vi "error_example.vi"() -> ()   [LabVIEW 2023, in "Error Handling Interface.lvlib" / "Error.lvclass"]
doc: "Demonstrates how to construct an error object and retrieve the log item from the class"
uses:
  Error.lvclass
  <vilib>/ActorFramework/Actor/Actor.lvclass
  Error.lvclass/Error.ctl
  create_displayable_msg.vi
  create_log_msg.vi
  error_type.ctl
panel:
  in  "error_mark":string="custom error message (error_mark)"
  in  "error_type":T1
  in  "error_to_process":errorcluster={"status"=TRUE, "code"=-550000, "source"="custom error range start"}
  out "error_msg_to_log":string
  out "error_msg_to_display":string
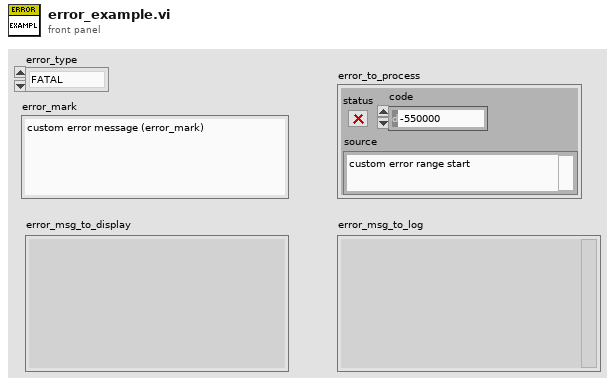
[diagram p1: front panel]
types:
  T1 = typedef "Error Handling Interface.lvlib/Error.lvclass/error_type.ctl" = enum16{"FATAL", "ERROR", "WARNING", "INFO", "DEBUG", "TRACE"}
  T2 = enum16{"none", "hifen", "fslash", "bslash", "vbar", "dot", "comma"}
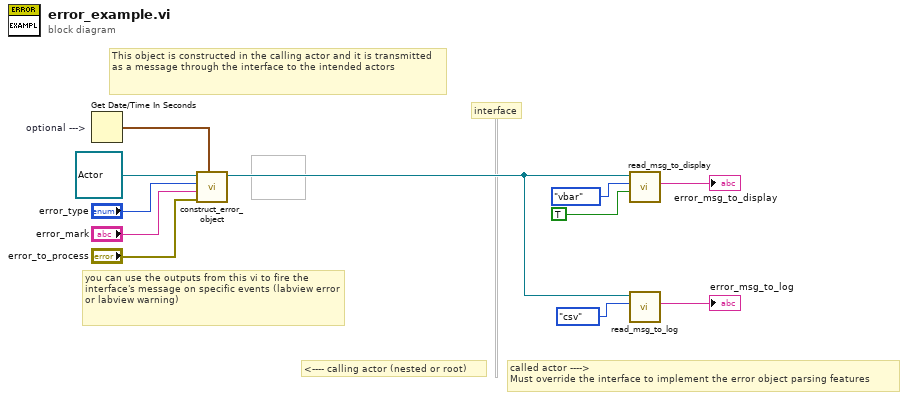
[diagram p0: block diagram]
diagram:
  # "you can use the outputs from this vi to fire the interface's message on specific events (labview error or labview warning)"
  # "interface"
  # "called actor ---->\nMust override the interface to implement the error object parsing features"
  # "<---- calling actor (nested or root)"
  # "This object is constructed in the calling actor and it is transmitted as a message through the interface to the intended actors"
  n1 = Get Date/Time In Seconds "optional --->"() -> (seconds since 1Jan1904=w11:timestamp)
  n2 = call "construct_error_object.vi"("error_time (now)"=w11, "error_to_process"="error_to_process", "error_mark"="error_mark", "error_type"="error_type", "error_source"=refnum<class "Actor.lvclass"> refnum ("Actor")) -> ("Error"=w2:refnum<class "Error.lvclass">)  [unwired: 4 in, 2 out]
  n3 = call "read_msg_to_display.vi"("pad_with_spaces (T)"=TRUE, "separator (none)"=T2."vbar", "Error in"=w2) -> ("error_msg_to_display"=→"error_msg_to_display":string)  [unwired: 8 in]
  n4 = call "read_msg_to_log.vi"("string_type (csv)"=enum16{"none", "csv", "json", "xml"}."csv" ("string_type"), "Error in"=w2) -> ("error_msg_to_log"=→"error_msg_to_log":string)  [unwired: 9 in]
